vi "Reset tracking.vi"(11 "Stop Tracking":T1(ring)) -> ()   [LabVIEW 2020]
uses:
  Global Variables/gl_UI Ctrl Refs.vi
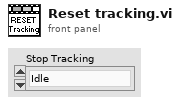
[diagram p1: front panel]
types:
  T1 = enum16{"Idle", "Stop Tracking", "Start Tracking"}
  T2 = typedef "UI ctrl refs cluster.ctl" = cluster{"Top level VI path":path, "Top level VI ref":refnum<vi>, "User menu ref":refnum<k9>, "Sub Panel control":refnum<vi>, "Imaging Param Tab":refnum<vi>, "Occurrence-Start drivers":refnum<k4>, "Occurrence-Speed logging initialised":refnum<k4>, "Occurrence-XYZ stage initialised":refnum<k4>, "Exit button":refnum<vi>, "Status ind":refnum<vi>, "Set as origin":refnum<vi>, "Speed Logging":refnum<vi>, "Time Lapse":refnum<vi>, "Live Imaging":refnum<vi>, "AOL Z Stack":refnum<vi>, "Motor Z Stack":refnum<vi>, "Funct Acq button":refnum<vi>, "Hard Shutter":refnum<vi>, "Virtual Shutter":refnum<vi>, "Laser Power":refnum<vi>, "AOL Mode":refnum<vi>, "Frame Size":refnum<vi>, "Field of View":refnum<vi>, "Dwell Time":refnum<vi>, "Zoom":refnum<vi>, "AOL Z":refnum<vi>, "Objective":refnum<vi>, "Axis":refnum<vi>, "Paths & Names":refnum<vi>, "Experiment folder path (ind.)":refnum<vi>, "Last State (Ind.)":refnum<vi>, "Averages":refnum<vi>, "Angle (degrees)":refnum<vi>, "X centre":refnum<vi>, "Y centre":refnum<vi>, "Plane Mode":refnum<vi>, "# Planes":refnum<vi>, "Z Start":refnum<vi>, "Z Stop":refnum<vi>, "Z Step":refnum<vi>, "PMT 1":refnum<vi>, "PMT 2":refnum<vi>, "Stage XYZ Position":refnum<vi>, "Pockels@Z Start":refnum<vi>, "Pockels@Z Stop":refnum<vi>, "Obtain Z Start":refnum<vi>, "Obtain Z Stop":refnum<vi>, "Live stim.trig.period":refnum<vi>, "Live stim.trig.enable":refnum<vi>, "Movement Correction":refnum<vi>, "Load Reference Image":refnum<vi>, "XY Stage Move":refnum<vi>, "MovCor Cluster":refnum<vi>, "RefDAQParam":refnum<vi>, "Funct. Acq. Pockels Modulation":refnum<vi>, "Ref Laser Power":refnum<vi>, "Enable Video Recording":refnum<vi>, "Video Record-Live Imaging":refnum<vi>, "Video Record-Funct acq":refnum<vi>, "Reference Source":refnum<vi>, "AOL Z-stack Chirps Ready (ind)":refnum<vi>, "Target time between mov.cor. ref triggers (ms)":refnum<vi>, "Funct. Acq. Ref frame save":refnum<vi>, "Tracking button":refnum<vi>, "Show ref plots window":refnum<vi>, "Center freq ind (nm)":refnum<vi>, "Pickup mode (ind)":refnum<vi>, "Logging queue (ind)":refnum<vi>, "Back aperture power (ind.)":refnum<vi>, "Power after objective (ind.)":refnum<vi>, "Switch user":refnum<vi>, "Ls1 Conn. Status":refnum<vi>, "Ls1Tuning Status":refnum<vi>, "Ls1 Faults":refnum<vi>, "Ls1 Connection":refnum<vi>, "Ls1 Mode":refnum<vi>, "Ls1 POWER [mW]":refnum<vi>, "Ls1Shutter":refnum<vi>, "Ls1 Wavelength":refnum<vi>, "Ls1 Note":refnum<vi>, "Ls1 Confirm Wav":refnum<vi>, "Ls1 PreChrp Prism1":refnum<vi>, "Ls1 PreChrp Prism2":refnum<vi>, "Ls1 wav top Ind":refnum<vi>, "Ls1 power top Ind":refnum<vi>, "Ls1 Pump peak Hold":refnum<vi>, "Ls1 Status Ind":refnum<vi>, "Ls1 wav cancel":refnum<vi>, "Experiment Type":refnum<vi>, "Biology Information":refnum<vi>, "Camera recording status":refnum<vi>}
  T3 = typedef "test_fpga_control.ctl" = cluster{"x_offset_host":fxp<+/-,16,8>, "y_offset_host":fxp<+/-,16,8>, "use host offset":bool, "Set_Ref_Centroid":bool, "OldChirpCode":bool, "use array of offsets":bool, "x_offset_host array":fxp<+/-,16,8>[], "y_offset_host array ":fxp<+/-,16,8>[], "use host offset Z":bool, "swap Z":bool, "z_offset_host ":fxp<+/-,16,8>}
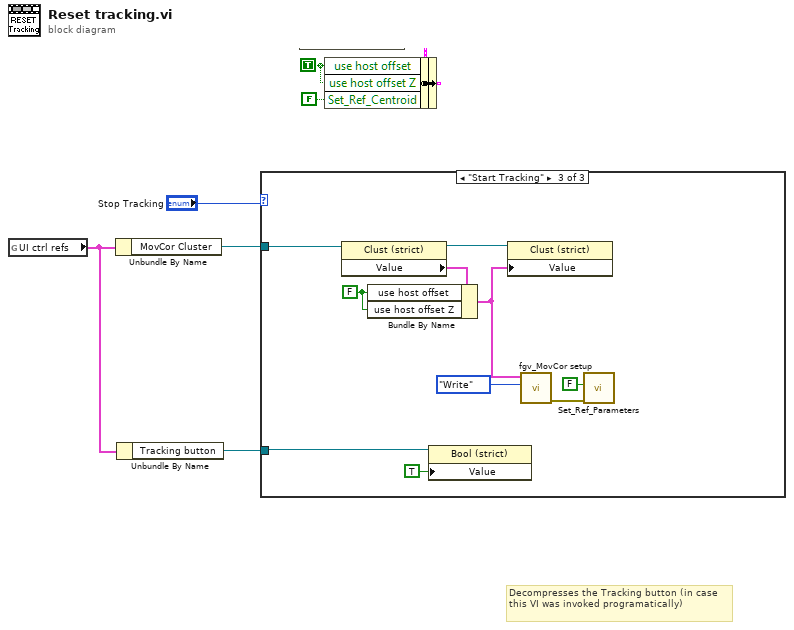
[diagram p0: block diagram]
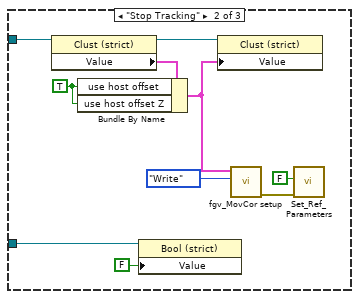
[diagram p3: hidden frame]
diagram:
  # "Decompresses the Tracking button (in case this VI was invoked programatically)"
  n1 = global read "gl_UI Ctrl Refs.vi" "UI ctrl refs"() -> (w2:T2)
  n2 = Unbundle By Name(w2) -> ("MovCor Cluster"=w4:refnum<vi>)
  n3 = Unbundle By Name(w2) -> ("Tracking button"=w3:refnum<vi>)
  n4 = case shown="\"Start Tracking\"" "Stop Tracking" {
    tunnel: w4 -> [_ w10 w16]
    tunnel: w3 -> [_ w7 w15]
    frame "Idle", Default {
    }
    frame "Stop Tracking" {
      w5 = TRUE ("use host offset")
      n5 = property on="Property Node" class="Clust (strict)"(reference=w10) -> (reference out=w12:refnum<vi>, "Value"=w11:T3)  [unwired: 1 in, 1 out]
      n6 = Bundle By Name(cluster=w11, "use host offset"=w5, "use host offset Z"=w5) -> (w13:T3)
      n7 = property on="Property Node" class="Bool (strict)"(reference=w7, "Value"=FALSE) -> ()  [unwired: 1 in, 2 out]
      n8 = property on="Property Node" class="Clust (strict)"(reference=w12, "Value"=w13) -> ()  [unwired: 1 in, 2 out]
      n9 = call "fgv_MovCor setup.vi"("Status"=enum16{"Initialize", "Write", "Read"}."Write", "MovCor Cluster"=w13) -> ("error out"=w8:errorcluster)  [unwired: 8 in, 1 out]
      n10 = call "Set_Ref_Parameters.vi"("error in"=w8, "use_increment_halfrate"=FALSE) -> ()  [unwired: 7 in, 3 out]
    }
    frame "Start Tracking" {
      w17 = FALSE ("use host offset")
      n11 = property on="Property Node" class="Clust (strict)"(reference=w16) -> (reference out=w22:refnum<vi>, "Value"=w21:T3)  [unwired: 1 in, 1 out]
      n12 = Bundle By Name(cluster=w21, "use host offset"=w17, "use host offset Z"=w17) -> (w23:T3)
      n13 = property on="Property Node" class="Bool (strict)"(reference=w15, "Value"=TRUE) -> ()  [unwired: 1 in, 2 out]
      n14 = property on="Property Node" class="Clust (strict)"(reference=w22, "Value"=w23) -> ()  [unwired: 1 in, 2 out]
      n15 = call "fgv_MovCor setup.vi"("Status"=enum16{"Initialize", "Write", "Read"}."Write", "MovCor Cluster"=w23) -> ("error out"=w19:errorcluster)  [unwired: 8 in, 1 out]
      n16 = call "Set_Ref_Parameters.vi"("error in"=w19, "use_increment_halfrate"=FALSE) -> ()  [unwired: 7 in, 3 out]
    }
  }
